vi "update file name.vi"(8 "error in":errorcluster, 11 "Video File in":refnum<class "Video File.lvclass">) -> (0 "error out":errorcluster, 3 "Video File out":refnum<class "Video File.lvclass">)   [LabVIEW 2023, in "File Classes.lvlib" / "Video File.lvclass"]
uses:
  Video File.lvclass
  D:/Library/LabVIEW Projects/Personal projects/Picture Organiser/PictureOrganizer/File Classes/File/File.lvclass
  Video File.lvclass/Video File.ctl
  File/File.lvclass/File.ctl
  File/Accessors/Read destination path.vi
  File/Accessors/Read file format.vi
  File/Read event name.vi
  File/Accessors/Read file extension.vi
  File/Accessors/Write new destination.vi
  File/File.lvclass
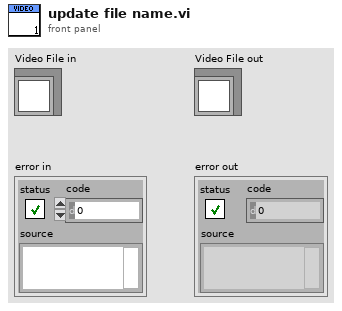
[diagram p1: front panel]
types:
  T1 = typedef "File Classes.lvlib/video exif info cluster.ctl" = cluster{"date":timestamp, "Model":string}
  T2 = enum16{"Date & Time (Default)", "Model Sufix", "Event Sufix", "Model & Event Sufix"}
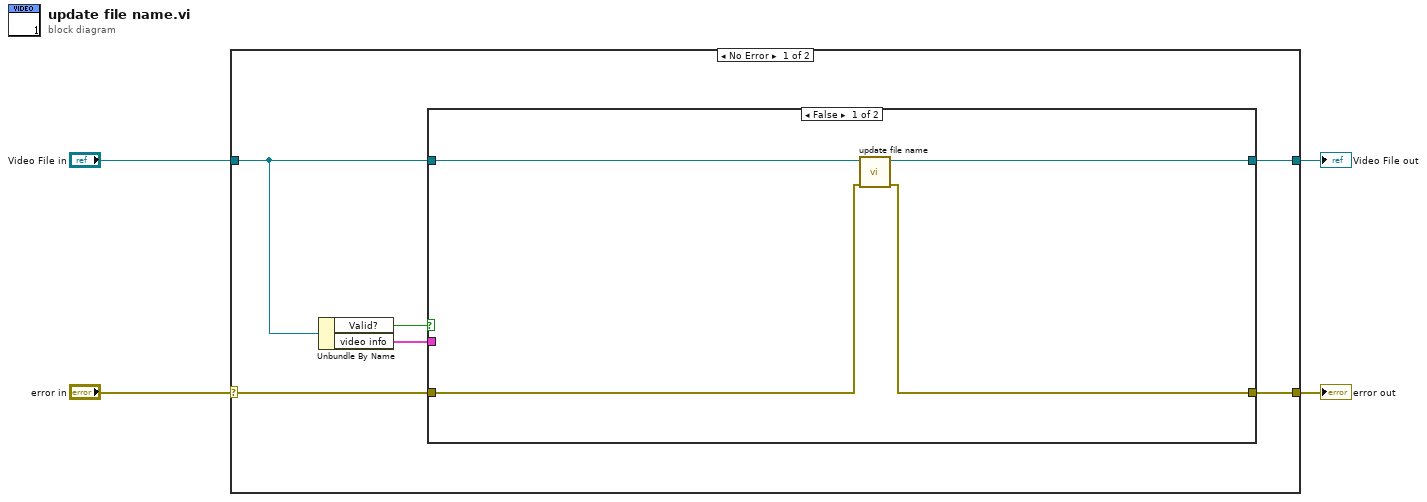
[diagram p0: block diagram]
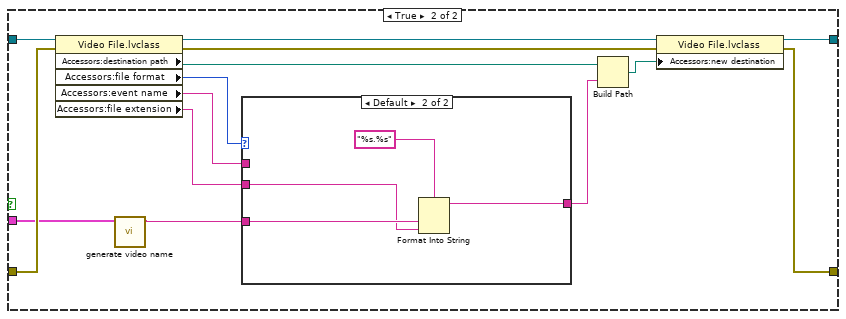
[diagram p2: hidden frame]
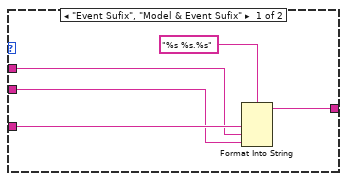
[diagram p3: hidden frame]
diagram:
  n1 = case shown="No Error" "error in" {
    selector: "error in" -> [w5 w39]
    tunnel: "Video File in" -> [w10 w38]
    tunnel: [w9 w38] -> w3
    tunnel: [w8 w39] -> w2
    frame No Error {
      n2 = Unbundle By Name(w10) -> ("Valid?"=w7:bool, "video info"=w6:T1)
      n3 = case shown="False" w7 {
        tunnel: [w14 w27] -> w9
        tunnel: w10 -> [w13 w28]
        tunnel: [w11 w18] -> w8
        tunnel: w5 -> [w12 w17]
        tunnel: w6 -> [_ w16]
        frame False {
          n4 = call-parent "update file name.vi"("error in (no error)"=w12, "File in"=w13) -> ("error out"=w11:errorcluster, "File out"=w14:refnum<class "Video File.lvclass">)  [unwired: 8 in]
        }
        frame True {
          n5 = property class="Video File.lvclass"(reference=w28, error in=w17) -> (reference out=w26:refnum<class "Video File.lvclass">, error out=w20:errorcluster, "Accessors:destination path"=w22:path, "Accessors:file format"=w23:T2, "Accessors:event name"=w25:string, "Accessors:file extension"=w24:string)
          n6 = call "generate video name.vi"("video info"=w16) -> ("date+model"=w15:string)  [unwired: 10 in]
          n7 = case shown="Default" w23 {
            tunnel: w25 -> [w30 _]
            tunnel: w24 -> [w29 w34]
            tunnel: [w32 w36] -> w19
            tunnel: w15 -> [w31 w35]
            frame "Event Sufix", "Model & Event Sufix" {
              n8 = Format Into String(format string="%s %s.%s" ("time format string (%c)"), w31, w30, w29) -> (resulting string=w32:string)  [unwired: 2 in, 1 out]
            }
            frame Default {
              n9 = Format Into String(format string="%s.%s" ("time format string (%c)"), w35, w34) -> (resulting string=w36:string)  [unwired: 2 in, 1 out]
            }
          }
          n10 = Build Path(base path=w22, name or relative path=w19) -> (appended path=w21:path)
          n11 = property class="Video File.lvclass"(reference=w26, error in=w20, "Accessors:new destination"=w21) -> (reference out=w27:refnum<class "Video File.lvclass">, error out=w18:errorcluster)
        }
      }
    }
    frame Error {
    }
  }
  "error out" <- w2
  "Video File out" <- w3
